vi "Init Msg Input.vi"(6 "Teller":refnum<class "Teller.lvclass">) -> (3 "Stop Msg Input out":refnum<class "Stop Msg Input.lvclass">)   [LabVIEW 2020, in "jettl.lvlib" / "Stop jettl Msg.lvlib" / "Stop Msg Input.lvlib" / "Stop Msg Input.lvclass"]
uses:
  Stop Msg Input.lvclass
  Teller/Teller.lvclass
  Stop Msg Input.lvclass/Stop Msg Input.ctl
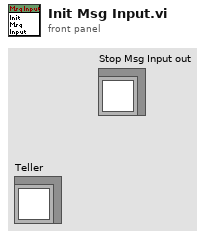
[diagram p1: front panel]
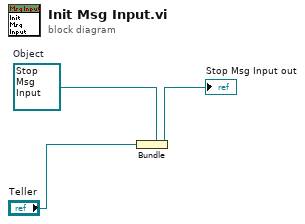
[diagram p0: block diagram]
diagram:
  w3 = refnum<class "Stop Msg Input.lvclass"> refnum  # Object
  n1 = Bundle "Bundle"(cluster=w3, "Teller") -> (→"Stop Msg Input out":refnum<class "Stop Msg Input.lvclass">)
